vi "FCE_TS_Action_PlotManager.vi"(8 "err in":errorcluster) -> (0 "err out":errorcluster)   [LabVIEW 2021]
uses:
  XLP80_FGlob/1886_FGlob_TDefs_Enum_FGlobItems.ctl
  XLP80_Globals/Globals_Settings_XLP80.vi
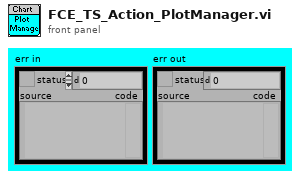
[diagram p1: front panel]
types:
  T1 = typedef "1886_FGlob_TDefs_Enum_FGlobItems.ctl" = enum16{"Put one", "Put all", "Recall one", "Recall all"}
  T2 = cluster{"LineStyle":u8[], "LineWidth":u8[], "LineColor":u32[], "SelectedPlot":i32[], "Scales":u16[], "Enabled":bool[]}
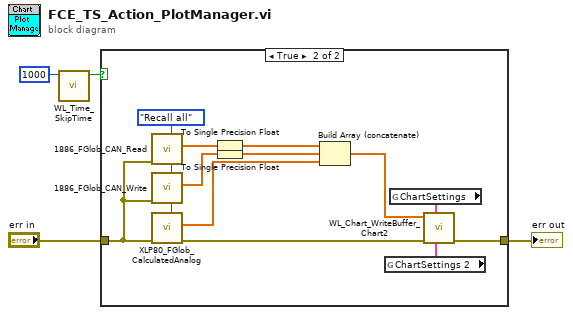
[diagram p0: block diagram]
diagram:
  n1 = call "WL_Time_SkipTime.vi"("SkipTime[ms]"=u32 1000) -> ("Run"=w3:bool)  [unwired: 9 in, 1 out]
  n2 = case shown="True" w3 {
    tunnel: [w5 w17] -> w1
    tunnel: "err in" -> [w5 w8]
    frame False {
    }
    frame True {
      w15 = 1886_FGlob_TDefs_Enum_FGlobItems."Recall all" ("Function (Recall One)")
      n3 = call "1886_FGlob_CAN_Read.vi"("Function (Recall One)"=w15, "err in"=w8) -> ("AI Values OUT"=w13:dbl[])  [unwired: 7 in, 2 out]
      n4 = call "1886_FGlob_CAN_Write.vi"("Function (Recall One)"=w15, "err in"=w8) -> ("AO Values OUT"=w12:dbl[])  [unwired: 7 in, 2 out]
      n5 = call "XLP80_FGlob_CalculatedAnalog.vi"("Function (Recall One)"=w15, "err in"=w8) -> ("err out"=w14:errorcluster, "Calc Values OUT"=w11:sgl[])  [unwired: 7 in, 1 out]
      n6 = To Single Precision Float(number=w13) -> (single precision float=w10:sgl[])
      n7 = To Single Precision Float(number=w12) -> (single precision float=w9:sgl[])
      n8 = Build Array (concatenate)(w10, w9, w11) -> (w16:sgl[])
      n9 = global read "Globals_Settings_XLP80.vi" "ChartSettings 2"() -> (w6:T2)
      n10 = global read "Globals_Settings_XLP80.vi" "ChartSettings"() -> (w7:T2)
      n11 = call "WL_Chart_WriteBuffer_Chart2.vi"("ChartSettings 2"=w6, "ChartSettings"=w7, "err in"=w14, "PlotValues"=w16) -> ("err out"=w17:errorcluster)  [unwired: 7 in]
    }
  }
  "err out" <- w1
